vi "Toggle DO State (manual mode).vi"(6 "ToggleInterval (250ms)":u32=250, 8 "error in (no error)":errorcluster, 9 "State":bool, 10 "DO IOName":string, 11 "DAQ":refnum<class "DAQ.lvclass">) -> (0 "error out":errorcluster, 3 "DAQ":refnum<class "DAQ.lvclass">)   [LabVIEW 2017, in "DAQ.lvclass"]
doc: "Developed by Kevin Thompson\nkevin@thompsonengineering.net\n\nCopyright 2018-2020\nThompson Engineering, LLC\nCall this Set DO State method for setting digital output states in test modules that are executed during automatic testing."
uses:
  DAQ.lvclass
  DataTypes/TD DAQ Output EventSenderMode-enum.ctl
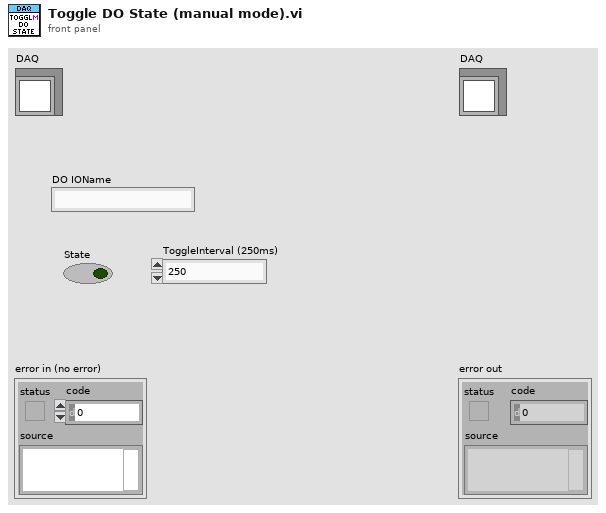
[diagram p1: front panel]
types:
  T1 = typedef "DAQ.lvclass/TD DAQ Output EventSenderMode-enum.ctl" = enum16{"manual", "automation"}
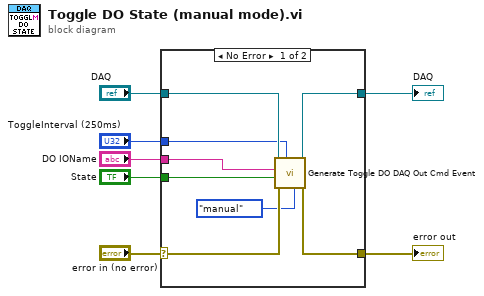
[diagram p0: block diagram]
diagram:
  n1 = case shown="No Error" "error in (no error)" {
    selector: "error in (no error)" -> [w15 w17]
    tunnel: [w14 w17] -> w6
    tunnel: [w12 w16] -> w4
    tunnel: "DAQ" -> [w13 w16]
    tunnel: "DO IOName" -> [w9 _]
    tunnel: "State" -> [w10 _]
    tunnel: "ToggleInterval (250ms)" -> [w8 _]
    frame No Error {
      n2 = call "Generate Toggle DO DAQ Out Cmd Event.vi"("mode (manual)"=TD_DAQ_Output_EventSenderMode-enum."manual" ("mode (automation)"), "ToggleInterval (250ms)"=w8, "error in (no error)"=w15, "BoolState"=w10, "DO IOName"=w9, "DAQ"=w13) -> ("error out"=w14:errorcluster, "DAQ"=w12:refnum<class "DAQ.lvclass">)  [unwired: 4 in]
    }
    frame Error {
    }
  }
  "error out" <- w6
  "DAQ" <- w4
